vi "bak.hReadChannels-UandP-2013.vi"(0 "FPGA VI Reference In":refnum<k20>, 1 "XYGraph Refnum":refnum<vi>, 3 "voltage out task":refnum<k21>, 4 "single channel voltage ref":refnum<vi>, 5 "Nsamples":u32=10000, 6 "error in":errorcluster, 7 "single channel array":refnum<vi>, 8 "voltage out error in":errorcluster, 10 "Tau/dt":sgl[](array[numeric]), 11 "Scale(mV)":sgl[](array[numeric]), 12 "single channel number":u32=15, 13 "voltage factor":dbl=100.0 format="%#_13g", 16 "SumScal":sgl[](array[numeric]), 17 "RawScal":sgl[](array[numeric]), 23 "offsets":sgl[](array[numeric])) -> (2 "Fehler":bool, 18 "task out":refnum<k21>, 19 "error out 2":errorcluster, 20 "FPGA VI Reference Out":refnum<k20>, 22 "PowerArray":sgl[][](array[numeric]), 25 "RawArray":sgl[][](array[numeric]), 26 "error out":errorcluster)   [LabVIEW 2014]
doc: "startet das einlesen und führt dies bis n Samples aus\nHier mit FIFO und IRQ."
uses:
  <vilib>/DAQmx/write.llb/DAQmx Write (Analog 1D DBL 1Chan NSamp).vi
  <vilib>/Utility/error.llb/Error Cluster From Error Code.vi
  <vilib>/rvi/errors/niLvFpgaAdjustHostInterfaceError.vi
  <vilib>/RVI Host/nirviSupport.llb/nirviErrorClusterFromErrorCode.vi
  <vilib>/DAQmx/miscellaneous.llb/DAQmx Fill In Error Info.vi
  <vilib>/rvi/interface/nirviReadWriteControl/nirviReadWriteControl.xnode
  FPGA Bitfiles/W7XBolo2017_FPGATarget_fmain2014_DACRangeVoltage.lvbitx
  f_main_2014.vi
  <vilib>/rvi/interface/nirviMethod/nirviMethod.xnode
  NiFpgaLv.dll
  <vilib>/rvi/interface/nirviMethod/StockFPGA_InlinedMethodWaitForMultipleIRQ.vi
  <vilib>/FPGAPlugInAG/PCI-7813R/niLvFpga_WaitOnIrq_PCI-7813R.vi
  <vilib>/FPGAPlugInAG/PCI-7813R/niLvFpga_AcknowledgeIrq_PCI-7813R.vi
  <vilib>/FPGAPlugInAG/PCI-7813R/niLvFpga_ReadFifo_PCI-7813R.vi
  <vilib>/rvi/errors/niLvFpgaMergeErrorWithErrorCode.vi
panel:
  in  "Tab Control":T1(tab)
  out "16bit integer voltage sample":i16[](array[numeric])
  out "XY Graph":cluster{"element":i64, "element":dbl}[](graph)
  out "Timed Out":bool
  out "STOP?":bool
  out "Elements Remaining":u32
  out "single channel voltage":sgl
  out "single channel voltage * factor":dbl
  out "empty sample array":dbl[](array[numeric])
  in  "Stop Voltage Output":bool
  out "single channel output error source":string
  out "Nsamples array":i64[](array[numeric])
  out "0th sample":sgl[](array[numeric])
  out "ScanID":u32
  out "canceled?":bool
  out "ScanID halt":bool
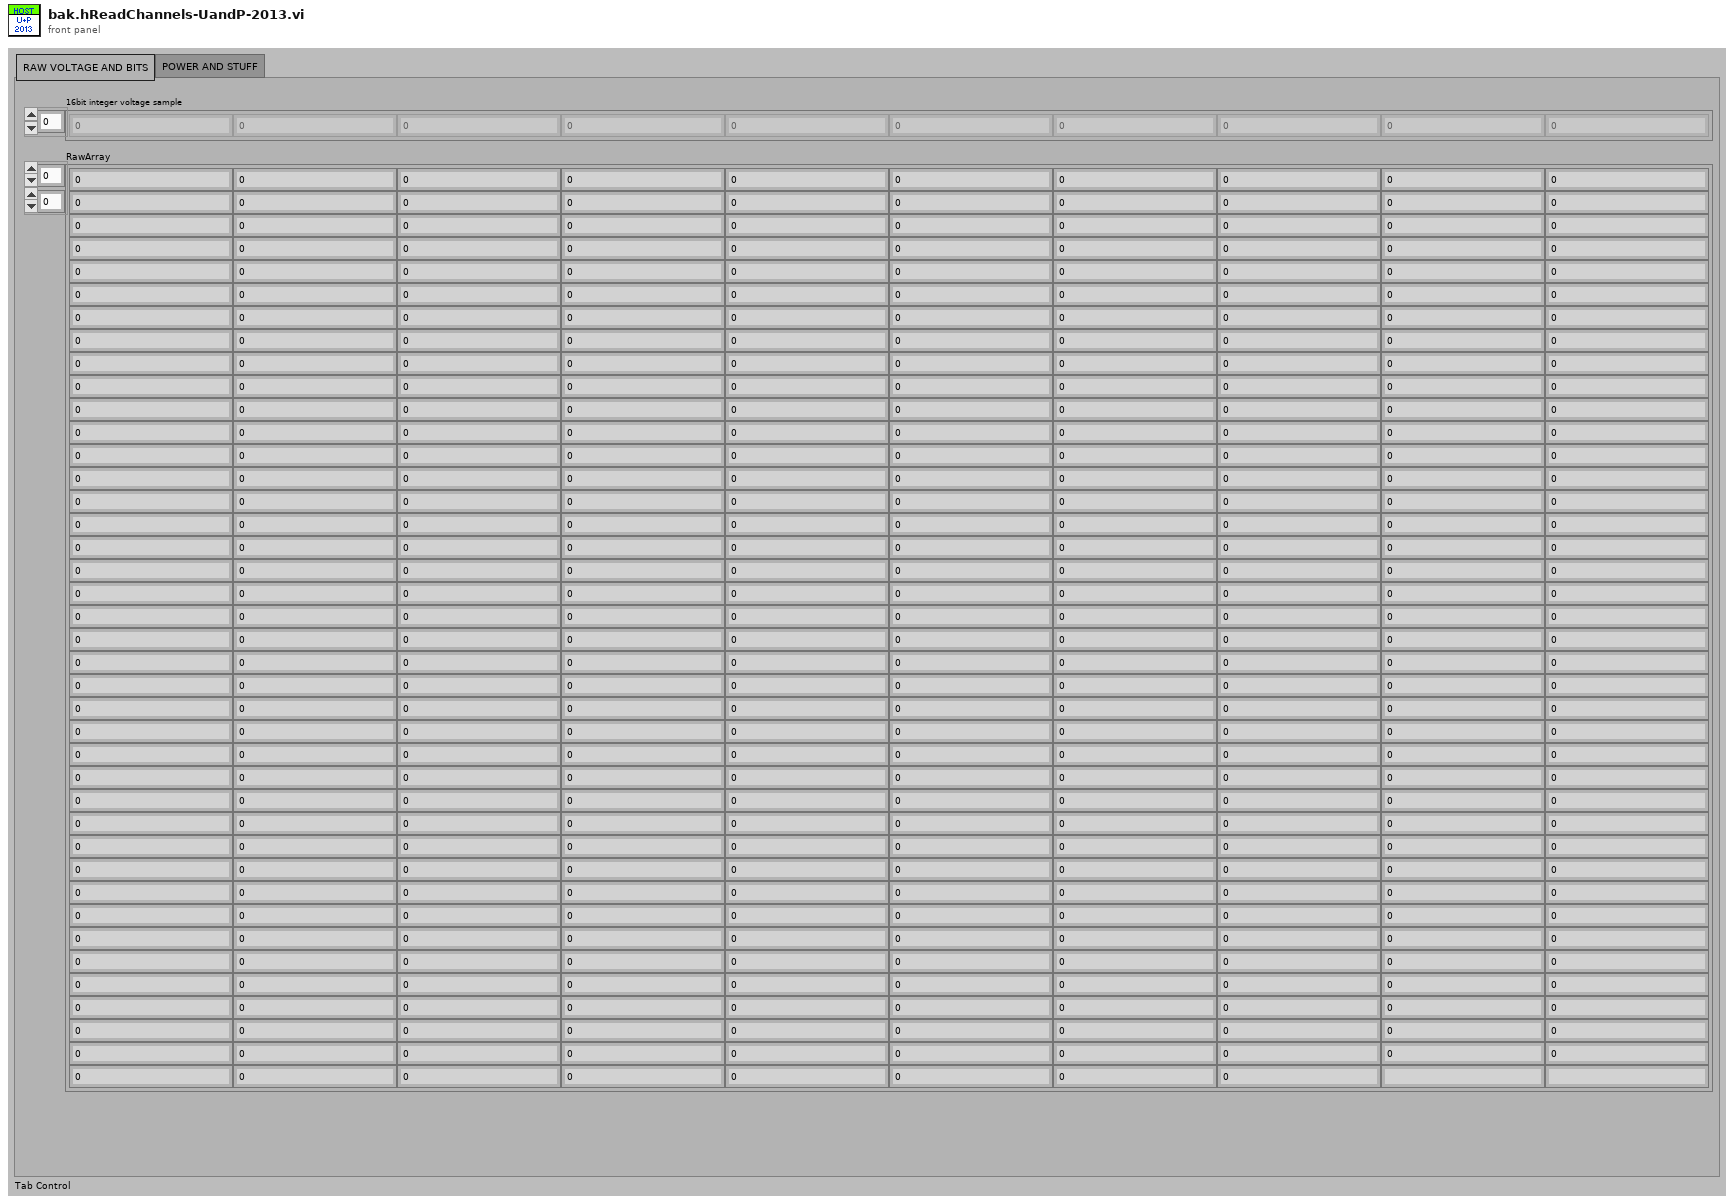
[diagram p1: front panel]
types:
  T1 = enum32{"RAW VOLTAGE AND BITS", "POWER AND STUFF"}
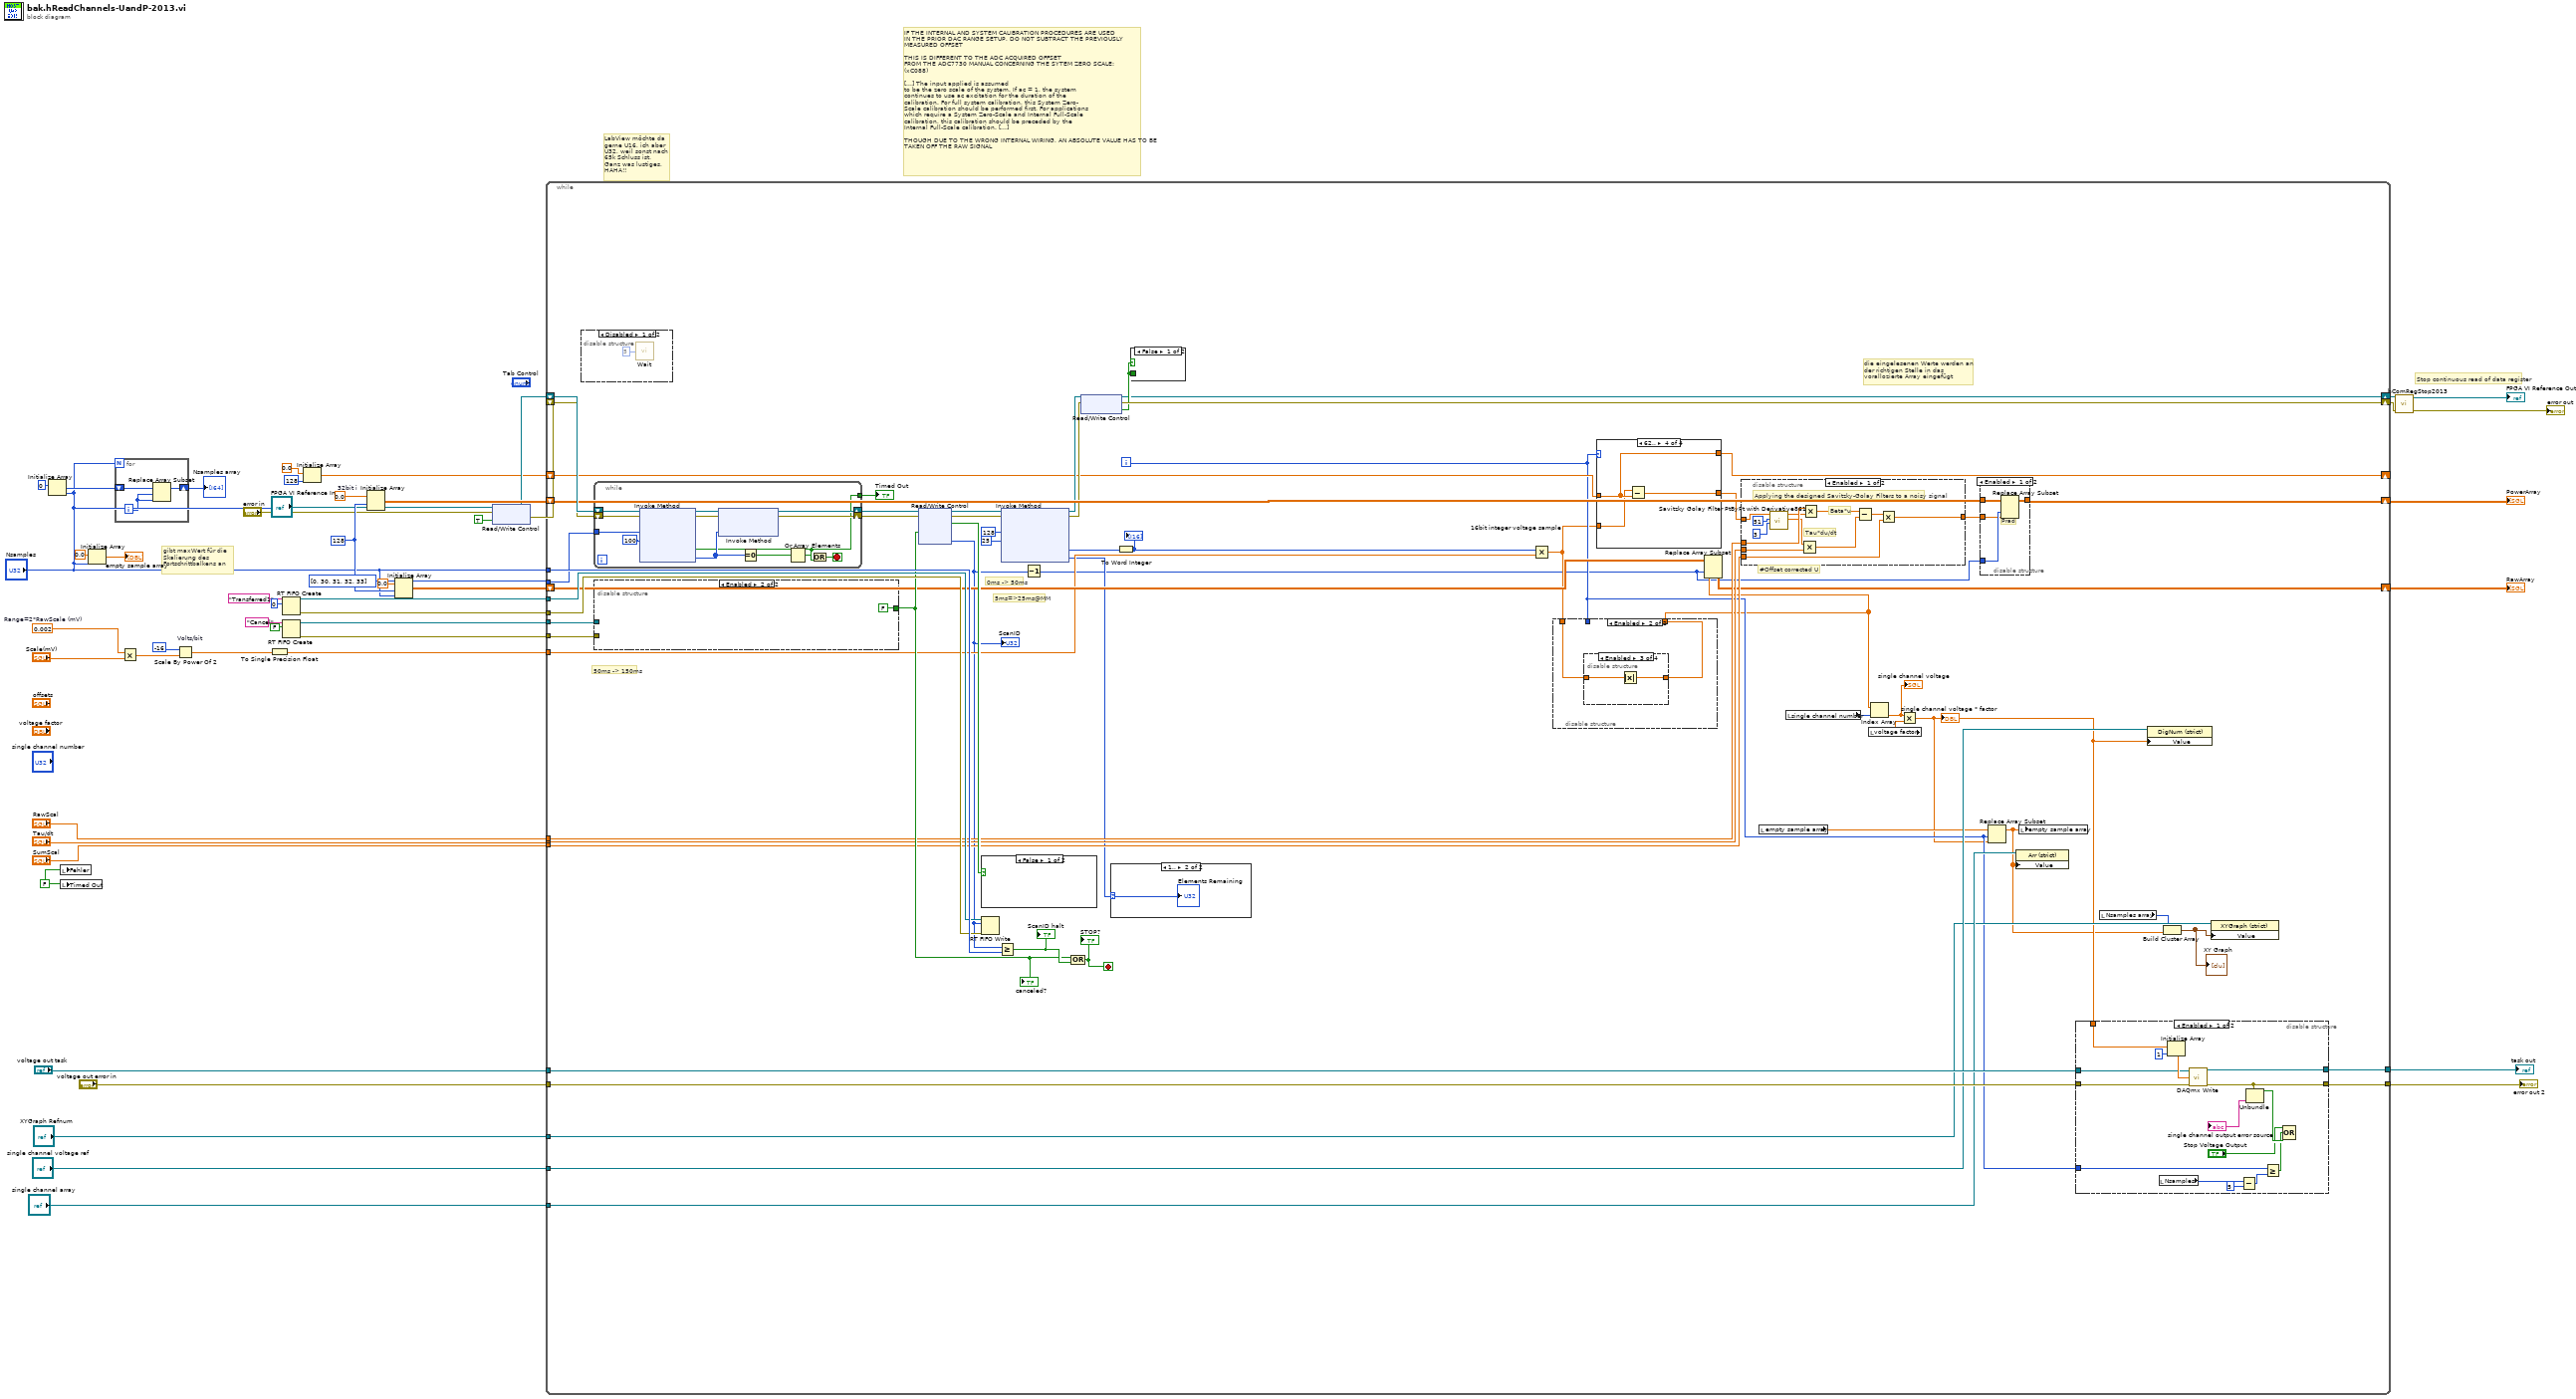
[diagram p0: block diagram]
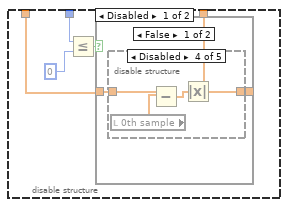
[diagram p2: hidden frame]
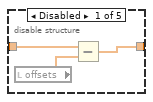
[diagram p3: hidden frame]
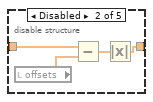
[diagram p4: hidden frame]
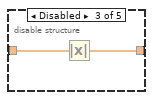
[diagram p5: hidden frame]
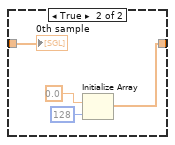
[diagram p7: hidden frame]
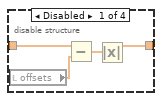
[diagram p8: hidden frame]
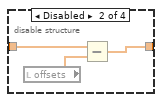
[diagram p9: hidden frame]
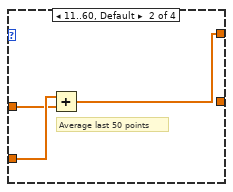
[diagram p15: hidden frame]
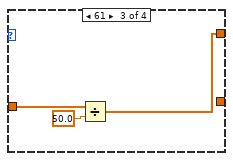
[diagram p16: hidden frame]
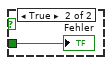
[diagram p17: hidden frame]
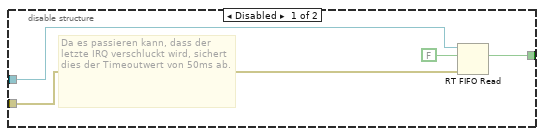
[diagram p18: hidden frame]
diagram:
  w6 = FALSE
  w25 = 0.002  # Range=2*RawScale (mV)
  w34 = 128 ("dimension size")
  w43 = sgl 0.0  # 32bit i
  # "IF THE INTERNAL AND SYSTEM CALIBRATION PROCEDURES ARE USED\nIN THE PRIOR DAC RANGE SETUP, DO NOT SUBTRACT THE PREVIOUSLY\nMEASURED OFFSET\n\nTHIS IS DIFFERENT TO THE ADC ACQUIRED OFFSET\nFROM THE ADC7730 MANUAL CONCERNING THE SYTEM ZERO SCALE:\n(xC088)\n\n[...] The input applied is assumed\nto be the zero scale of the system. If ac = 1, the system\ncontinues to use ac excitation for the duration of the\ncalibration. For full system calibration, this System Zero-\nScale calibration should be performed first. For applications\nwhich require a System Zero-Scale and Internal Full-Scale\ncalibration, this calibration should be preceded by the\nInternal Full-Scale calibration. [...]\n\nTHOUGH DUE TO THE WRONG INTERNAL WIRING, AN ABSOLUTE VALUE HAS TO BE\nTAKEN OFF THE RAW SIGNAL"
  # "Stop continuous read of data register"
  # "gibt maxWert für die Skalierung des Fortschrittbalkens an"
  # "LabView möchte da gerne U16, ich aber U32, weil sonst nach 65k Schluss ist. \nGanz was lustiges, HAHA!!"
  n1 = Initialize Array(i64 0 ("element"), "Nsamples") -> (w9:i64[])
  n2 = local write "Fehler"(w6) -> ()
  n3 = local write "Timed Out"(w6) -> ()
  n4 = Initialize Array(0.0 ("element"), "Nsamples") -> (→"empty sample array":dbl[])
  n5 = for {
    N: "Nsamples" -> [_]
    shift-right: [w52] -> w8
    shift-left: w9 -> [w54]
    i -> [w53]
    n6 = Replace Array Subset(array=w54, new element=w53, index=w53) -> (w52:i64[])
  }
  "Nsamples array" <- w8
  n7 = Multiply(x=w25, y="Scale(mV)") -> (x*y=w26:dbl[])
  n8 = Scale By Power Of 2 "Volts/bit"(n=i16 -16, x=w26) -> (x*2^n=w27:dbl[])
  n9 = To Single Precision Float(number=w27) -> (single precision float=w24:sgl[])
  n10 = RT FIFO Create(0:"Transferred1" ("name (unnamed)"), 1:u32 0) -> (8:w48:refnum<k33>, 11:w47:errorcluster)  [unwired: 2 in, 5 out]
  n11 = RT FIFO Create(0:"Cancel" ("name (unnamed)"), 1:FALSE) -> (8:w45:refnum<k33>, 11:w44:errorcluster)  [unwired: 2 in, 5 out]
  n12 = Initialize Array(sgl 0.0 ("element"), 128 ("dimension size")) -> (w17:sgl[])
  n13 = Initialize Array(w43, w34, "Nsamples") -> (w42:sgl[][])
  n14 = Initialize Array(sgl 0.0, w34, "Nsamples") -> (w51:sgl[][])
  n15 = xnode "Read/Write Control"("FPGA VI Reference In"="FPGA VI Reference In", "error in"="error in", "ADCRead"=TRUE) -> ("FPGA VI Reference Out"=w31:refnum<k20>, "error out"=w30:errorcluster)
  n16 = while {
    tunnel: "Nsamples" -> [w108]
    shift-right: [w71] -> w35
    shift-left: w51 -> [w98]
    shift-right: [w69] -> w41
    shift-left: w31 -> [w111]
    shift-right: [w109] -> w40
    shift-left: w30 -> [w110]
    tunnel: w48 -> [w107]
    tunnel: w47 -> [w106]
    tunnel: w45 -> [w104]
    tunnel: w44 -> [w103]
    shift-right: [w70] -> w36
    shift-left: w42 -> [w102]
    tunnel: w24 -> [w97]
    tunnel: "Tau/dt" -> [w94]
    tunnel: "SumScal" -> [w96]
    tunnel: "RawScal" -> [w95]
    shift-right: [w87] -> _
    shift-left: w17 -> [w86]
    tunnel: i32[] [0, 30, 31, 32, 33] -> [w81]
    tunnel: "voltage out task" -> [w78]
    tunnel: "voltage out error in" -> [w77]
    tunnel: [w76] -> w3
    tunnel: [w75] -> w2
    tunnel: "single channel array" -> [w74]
    tunnel: "single channel voltage ref" -> [w73]
    tunnel: "XYGraph Refnum" -> [w72]
    i -> [w68]
    stop <- w82 stop-if-true
    # "#Offset corrected U"
    # "5ms=>25ms@MM"
    # "0ms -> 50ms"
    # "50ms -> 150ms"
    # "die eingelesenen Werte werden an der richtigen Stelle in das vorallozierte Array eingefügt"
    n17 = disable-structure shown="Disabled" {
      frame Disabled {
        n18 = call "Wait"("Count(uSec)"=u32 5) -> ()  [unwired: 1 out]
      }
      frame Enabled {
      }
    }
    n19 = while {
      tunnel: [w197] -> w85
      shift-right: [w199] -> w79
      shift-left: w111 -> [w206]
      shift-right: [w198] -> w80
      shift-left: w110 -> [w205]
      tunnel: w81 -> [w203]
      stop <- w196 stop-if-true
      n20 = xnode "Invoke Method"("FPGA VI Reference In"=w206, "error in"=w205, "IRQ Number(s)"=w203, "Timeout (ms)"=100) -> ("FPGA VI Reference Out"=w200:refnum<k20>, "error out"=w201:errorcluster, "Timed Out"=w197:bool, "IRQ(s) Asserted"=w202:i32[])
      n21 = xnode "Invoke Method"("FPGA VI Reference In"=w200, "error in"=w201, "IRQ Number(s)"=w202) -> ("FPGA VI Reference Out"=w199:refnum<k20>, "error out"=w198:errorcluster)
      n22 = Equal To 0?(x=w202) -> (x = 0?=w195:bool[])
      n23 = Or Array Elements(Boolean array=w195) -> (logical OR=w194:bool)
      n24 = Or(x=w194, y=w197) -> (x .or. y?=w196:bool)
    }
    "Timed Out" <- w85
    n25 = disable-structure shown="Enabled" {
      disable-tunnel: [w211 FALSE] -> w105
      disable-tunnel: w104 -> [w210 _]
      disable-tunnel: w103 -> [w209 _]
      frame Disabled {
        # "Da es passieren kann, dass der letzte IRQ verschluckt wird, sichert dies der Timeoutwert von 50ms ab."
        n26 = RT FIFO Read(0:w210, 1:FALSE ("element"), 3:w209) -> (9:w211:bool)  [unwired: 5 out]
      }
      frame Enabled {
      }
    }
    "canceled?" <- w105
    n27 = xnode "Read/Write Control"("FPGA VI Reference In"=w79, "error in"=w80, "cancel"=w105) -> ("FPGA VI Reference Out"=w100:refnum<k20>, "error out"=w99:errorcluster, "Timeout"=w101:bool, "ScanID"=w55:u32)
    "ScanID" <- w55
    n28 = case shown="False" w101 {
      selector: w101 -> [_ w215]
      frame False {
      }
      frame True {
        n29 = local write "Fehler"(w215) -> ()
      }
    }
    n30 = RT FIFO Write(0:w107, 1:w55, 3:w106) -> ()  [unwired: 1 in, 5 out]
    n31 = Greater Or Equal?(x=w55, y=w108) -> (x >= y?=w112:bool)
    "ScanID halt" <- w112
    n32 = xnode ("Invoke Method")("FPGA VI Reference In"=w100, "error in"=w99, "Number of Elements"=u32 128, "Timeout (ms)"=25 ("Timeout")) -> ("FPGA VI Reference Out"=w89:refnum<k20>, "error out"=w88:errorcluster, "Data"=w91:u32[], "Elements Remaining"=w84:u32)
    n33 = Decrement(x=w55) -> ()  [unwired: 1 out]
    n34 = Compound Arithmetic op=OR(w105, w112) -> (w82:bool)
    "STOP?" <- w82
    n35 = xnode "Read/Write Control"("FPGA VI Reference In"=w89, "error in"=w88) -> ("FPGA VI Reference Out"=w69:refnum<k20>, "error out"=w109:errorcluster, "Fifo-Fehler"=w83:bool)
    n36 = case shown="1.." w84 {
      selector: w84 -> [_ w213]
      frame 0, Default {
      }
      frame 1.. {
        "Elements Remaining" <- w213
      }
    }
    n37 = To Word Integer(number=w91) -> (16bit integer=w90:i16[])
    "16bit integer voltage sample" <- w90
    n38 = case shown="False" w83 {
      tunnel: w83 -> [_ w207]
      frame False {
      }
      frame True {
        "Fehler" <- w207
      }
    }
    n39 = Multiply(x=w90, y=w97) -> (x*y=w57:sgl[])
    n40 = disable-structure shown="Enabled" {
      disable-tunnel: w68 -> [w117 _]
      disable-tunnel: w57 -> [w114 w139]
      disable-tunnel: [w113 w138] -> w56
      frame Disabled {
        n41 = Less Or Equal?(x=w117, y=0) -> (x <= y?=w115:bool)
        n42 = case shown="False" w115 {
          tunnel: w114 -> [w119 w134]
          tunnel: [w118 w135] -> w113
          frame False {
            n43 = disable-structure shown="Disabled" {
              disable-tunnel: w119 -> [w122 w126 w128 w130 w133]
              disable-tunnel: [w120 w123 w127 w131 w133] -> w118
              frame Disabled {
                n44 = local read "offsets"() -> (w121:sgl[])
                n45 = Subtract(x=w122, y=w121) -> (x-y=w120:sgl[])
              }
              frame Disabled {
                n46 = local read "offsets"() -> (w125:sgl[])
                n47 = Subtract(x=w126, y=w125) -> (x-y=w124:sgl[])
                n48 = Absolute Value(x=w124) -> (abs(x)=w123:sgl[])
              }
              frame Disabled {
                n49 = Absolute Value(x=w128) -> (abs(x)=w127:sgl[])
              }
              frame Disabled {
                n50 = local read "0th sample"() -> (w129:sgl[])
                n51 = Subtract(x=w130, y=w129) -> (x-y=w132:sgl[])
                n52 = Absolute Value(x=w132) -> (abs(x)=w131:sgl[])
              }
              frame Enabled {
              }
            }
          }
          frame True {
            n53 = Initialize Array(sgl 0.0 ("element"), 128 ("dimension size")) -> (w135:sgl[])
            "0th sample" <- w134
          }
        }
      }
      frame Enabled {
        n54 = disable-structure shown="Enabled" {
          disable-tunnel: w139 -> [w142 w145 w147 w148]
          disable-tunnel: [w140 w143 w146 w148] -> w138
          frame Disabled {
            n55 = local read "offsets"() -> (w141:sgl[])
            n56 = Subtract(x=w142, y=w141) -> (x-y=w140:sgl[])
            n57 = Absolute Value(x=w140) -> ()  [unwired: 1 out]
          }
          frame Disabled {
            n58 = local read "offsets"() -> (w144:sgl[])
            n59 = Subtract(x=w145, y=w144) -> (x-y=w143:sgl[])
          }
          frame Enabled {
            n60 = Absolute Value(x=w147) -> (abs(x)=w146:sgl[])
          }
          frame Disabled {
          }
        }
      }
    }
    n61 = case shown="62.." w68 {
      tunnel: w57 -> [_ w186 _ w192]
      tunnel: [w184 w187 w189 w193] -> w87
      tunnel: w86 -> [w184 w185 w190 w193]
      tunnel: [w184 _ _ w191] -> w66
      frame 0..10 {
      }
      frame 11..60, Default {
        # "Average last 50 points"
        n62 = Add(x=w186, y=w185) -> (x+y=w187:sgl[])
      }
      frame 61 {
        n63 = Divide(x=w190, y=sgl 50.0) -> (x/y=w189:sgl[])
      }
      frame 62.. {
        n64 = Subtract(x=w192, y=w193) -> (x-y=w191:sgl[])
      }
    }
    n65 = Replace Array Subset(array=w98, new element=w56, index (col)=w55) -> (w71:sgl[][])  [unwired: 1 in]
    n66 = disable-structure shown="Enabled" {
      disable-tunnel: w96 -> [w182 _]
      disable-tunnel: w95 -> [w181 _]
      disable-tunnel: w94 -> [w180 _]
      disable-tunnel: [w179 w183] -> w67
      disable-tunnel: w66 -> [w178 w183]
      frame Enabled {
        # "Beta*u"
        # "Tau*du/dt"
        # "Applying the designed Savitzky-Golay Filters to a noisy signal"
        n67 = call "Savitzky Golay Filter PtByPt with Derivative861.vi"("order polynomial"=3, "side points"=51, "x"=w178) -> ("Filtered Derivative"=w174:dbl[], "Filtered x"=w175:dbl[])  [unwired: 1 in, 6 out]
        n68 = Multiply(x=w174, y=w180) -> (x*y=w173:dbl[])
        n69 = Multiply(x=w181, y=w175) -> (x*y=w177:dbl[])
        n70 = Subtract(x=w177, y=w173) -> (x-y=w176:dbl[])
        n71 = Multiply(x=w176, y=w182) -> (x*y=w179:dbl[])
      }
      frame Disabled {
      }
    }
    n72 = local read "empty sample array"() -> (w63:dbl[])
    n73 = local read "single channel number"() -> (w65:u32)
    n74 = local read "voltage factor"() -> (w64:dbl)
    n75 = Index Array(array=w56, index=w65) -> (element=w62:sgl)
    "single channel voltage" <- w62
    n76 = Multiply(x=w62, y=w64) -> (x*y=w61:dbl)
    "single channel voltage * factor" <- w61
    n77 = disable-structure shown="Enabled" {
      disable-tunnel: w102 -> [w169 w170]
      disable-tunnel: [w168 w170] -> w70
      disable-tunnel: w55 -> [w167 _]
      disable-tunnel: w67 -> [w166 _]
      frame Enabled {
        # "Prad"
        n78 = Replace Array Subset(array=w169, new element=w166, index (col)=w167) -> (w168:sgl[][])  [unwired: 1 in]
      }
      frame Disabled {
      }
    }
    n79 = Replace Array Subset(array=w63, new element=w61, index=w68) -> (w60:dbl[])
    n80 = property class="Arr (strict)"(reference=w74, "Value"=w60) -> ()  [unwired: 1 in, 2 out]
    n81 = local write "empty sample array"(w60) -> ()
    n82 = disable-structure shown="Enabled" {
      disable-tunnel: w68 -> [w158 _]
      disable-tunnel: w78 -> [w157 w165]
      disable-tunnel: w77 -> [w156 w164]
      disable-tunnel: [w155 w165] -> w76
      disable-tunnel: [w154 w164] -> w75
      disable-tunnel: w61 -> [w153 _]
      frame Enabled {
        n83 = local read "Nsamples"() -> (w151:u32)
        n84 = Initialize Array(w153, 1 ("dimension size")) -> (w163:dbl[])
        n85 = call-poly <vilib>:"DAQmx Write.vi"("task/channels in"=w157, "data"=w163, "error in"=w156) -> ("task out"=w155:refnum<k21>, "error out"=w154:errorcluster)  [unwired: 10 in, 1 out]
        n86 = Subtract(x=w151, y=u32 5) -> (x-y=w149:u32)
        n87 = Unbundle(w154) -> ("status"=w161:bool, "source"=→"single channel output error source":string)  [unwired: 1 out]
        n88 = Greater Or Equal?(x=w158, y=w149) -> (x >= y?=w160:bool)
        n89 = Compound Arithmetic op=OR("Stop Voltage Output", w160, w161) -> ()  [unwired: 1 out]
      }
      frame Disabled {
      }
    }
    n90 = local read "Nsamples array"() -> (w59:i64[])
    n91 = property class="DigNum (strict)"(reference=w73, "Value"=w61) -> ()  [unwired: 1 in, 2 out]
    n92 = Build Cluster Array(w59, w60) -> (w58:cluster{"element":i64, "element":dbl}[])
    "XY Graph" <- w58
    n93 = property class="XYGraph (strict)"(reference=w72, "Value"=w58) -> ()  [unwired: 1 in, 2 out]
  }
  "RawArray" <- w35
  "PowerArray" <- w36
  "task out" <- w3
  "error out 2" <- w2
  n94 = call "hComRegStop2013.vi"("error in"=w40, "FPGA VI Reference In"=w41) -> ("error out"=→"error out":errorcluster, "FPGA VI Reference Out"=→"FPGA VI Reference Out":refnum<k20>)  [unwired: 3 in, 1 out]
